vi "setBuffer.vi"(10 "Buffer":u16[](array[numeric]), 11 "ModbusBuffer in":refnum<class "ModbusBufferBuilder.lvclass">) -> (3 "ModbusBuffer out":refnum<class "ModbusBufferBuilder.lvclass">)   [LabVIEW 2016, in "ModbusBufferBuilder.lvclass"]
uses:
  ModbusBufferBuilder.lvclass
  ModbusBufferBuilder.lvclass/ModbusBufferBuilder.ctl
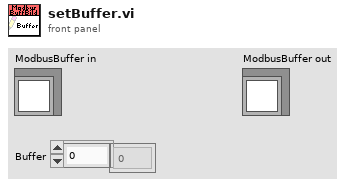
[diagram p1: front panel]
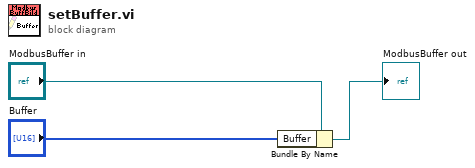
[diagram p0: block diagram]
diagram:
  n1 = Bundle By Name(cluster="ModbusBuffer in", "Buffer"="Buffer") -> (→"ModbusBuffer out":refnum<class "ModbusBufferBuilder.lvclass">)
